vi "gaussian FWHM to w0.vi"(11 "FWHM":dbl) -> (3 "w0":dbl)   [LabVIEW 2020]
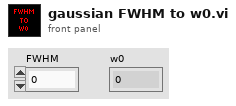
[diagram p1: front panel]
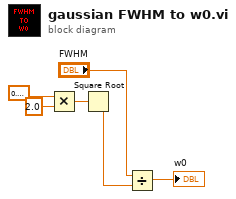
[diagram p0: block diagram]
diagram:
  n1 = Multiply(x=0.6931471805599453, y=2.0) -> (x*y=w1:dbl)
  n2 = Square Root(x=w1) -> (sqrt(x)=w5:dbl)
  n3 = Divide(x="FWHM", y=w5) -> (x/y=→"w0":dbl)
